vi "init_scope.vi"(8 "error in (no error)":errorcluster, 10 "VISA Timeout (millis)":u32=30000, 11 "VISA Scope":refnum<visa-resource-name>) -> (0 "error out":errorcluster, 3 "VISA Scope Out":refnum<visa-resource-name>)   [LabVIEW 2011]
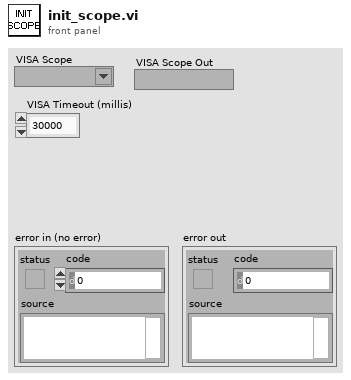
[diagram p1: front panel]
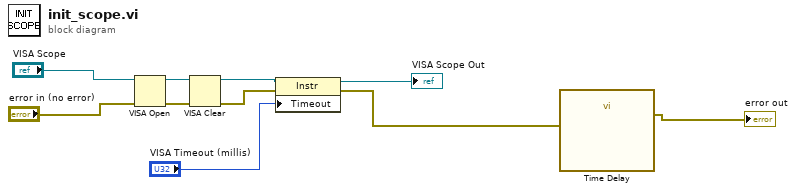
[diagram p0: block diagram]
diagram:
  n1 = VISA Open(error in (no error)="error in (no error)", VISA resource name="VISA Scope") -> (VISA resource name=w7:refnum<visa-resource-name>, error out=w8:errorcluster)  [unwired: 3 in]
  n2 = VISA Clear(VISA resource name=w7, error in (no error)=w8) -> (VISA resource name out=w6:refnum<visa-resource-name>, error out=w5:errorcluster)
  n3 = property class="Instr"(reference=w6, error in=w5, "Timeout"="VISA Timeout (millis)") -> (reference out=→"VISA Scope Out":refnum<visa-resource-name>, error out=w2:errorcluster)
  n4 = call "Time Delay"("error in (no error)"=w2) -> ("error out"=→"error out":errorcluster)  [unwired: 10 in]
